vi "Switch Pulser.vi"(1 "Boolean":bool) -> (0 "Boolean 2":bool)   [LabVIEW 2014]
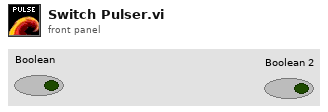
[diagram p1: front panel]
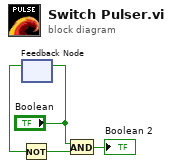
[diagram p0: block diagram]
diagram:
  n1 = feedback-in #1("Boolean") -> ()
  n2 = feedback #1() -> (w3:bool)  [unwired: 1 in]
  n3 = Not(x=w3) -> (.not. x?=w4:bool)
  n4 = And(x="Boolean", y=w4) -> (x .and. y?=→"Boolean 2":bool)
